vi "Write DAQ FIFO.vi"(6 "FIFO Timestamps":T2, 8 "error in (no error)":errorcluster, 9 "Timeout (ms)":i32, 10 "Data In":T1[](array[typedef]), 11 "CIFFIFO in":refnum<class "CIF_CIPC_Fifo_DAQ.lvclass">) -> (0 "error out":errorcluster, 1 "timed out?":bool, 2 "Data Out":T1[](array[typedef]), 3 "CIFFIFO out":refnum<class "CIF_CIPC_Fifo_DAQ.lvclass">)   [LabVIEW 2021, in "CIF_CIPC_Fifo_DAQ.lvclass"]
uses:
  CIF_CIPC_Fifo_DAQ.lvclass
  ChannelCommon/typedef/TimeStamps.ctl
  D:/dev/Packages/CIF_Channels_Core/src/CIPC_Channels/CIF_CIPC_Chan/CIF_CIPC_Chn.lvclass
  D:/dev/Packages/CIF_Channels_Core/src/CIFChannels/CIFChannels.lvclass
  ChannelCommon/typedef/Datatype Waveform.ctl
  CIFChannels/CIFChannels.lvclass/CIFChannels.ctl
  CIF_CIPC_Chan/CIF_CIPC_Chn.lvclass/CIF_CIPC_Chn.ctl
  <vilib>/CIF Foundation/CIF Utilities/Statistics/I64/Stats_I64_CIF_U.lvclass/Stats_I64_CIF_U.ctl
  CIF_CIPC_Chan/Accessors/Read Buffer Configuration.vi
  CIF_CIPC_Chan/SubVIs/Check Writer Backpressure.vi/7796537b-0e69-421b-96bb-30a861203fb6.vi
  CIFChannels/Accessors/Read FIFO Backpressure.vi
  CIFChannels/Utilities/Update Channel Benchmark.vi
  SubVIs/Core Write DAQ FIFO.vi/1bad10da-a98b-49ee-b03a-18b497e396df.vi
  SubVIs/Core Write DAQ FIFO.vi/70f860b1-5d4a-43dc-b0c2-c9446e8447f7.vi
  CIF_CIPC_Chan/Accessors/Read CIPC Channel.vi
  SubVIs/Write One DAQ Waveform.vi
  CIFChannels/Utilities/Create Flattened FIFO Header.vi
  CIF_CIPC_Chan/SubVIs/Write FIFO Header to CIPC.vi/2516c5c4-bcd6-4eab-a054-fa3d4f1376bc.vi
  CIF_CIPC_Chan/SubVIs/Check Writer Backpressure.vi/7796537b-0e69-421b-96bb-30a861203fb6.vi/3d5c1244-b460-4622-96d1-ee1e369932ac.vi
  <vilib>/CIF Foundation/CIF CIPC/Utilities/Get Size.vi
  CIF_CIPC_Chan/SubVIs/Check Writer Backpressure.vi/7796537b-0e69-421b-96bb-30a861203fb6.vi/b3361ac9-0b85-4d75-8feb-76d028d0c03f.vi
  <vilib>/CIF Foundation/CIF CIPC/SubVIs/Get Element Write Position.vi
  <vilib>/CIF Foundation/CIF Utilities/Statistics/I64/X1 minus X0.vi
  <vilib>/CIF Foundation/CIF Utilities/Time/System Time/Get System Time.vi
  SubVIs/Write One DAQ Waveform.vi/48238f55-1c09-49b5-9564-fcee243396a4.vi
  SubVIs/Write One DAQ Waveform.vi/652cb35b-0a2d-4ac6-8d88-471c3b57ed63.vi
  SubVIs/Write One DAQ Waveform.vi/5604da8b-43be-42ee-b0d1-5bd59e62de3d.vi
  SubVIs/Write One DAQ Waveform.vi/489ce88f-d13b-4e3d-8a44-beac6fbb575f.vi
  ChannelCommon/Utilities/Flatten Header.vi
  CIFChannels/Utilities/Update FIFO Header.vi
  ChannelCommon/Utilities/Add Header Bytes.vi
  <vilib>/CIF Foundation/CIF CIPC/SubVIs/Check Error.vi
  <vilib>/CIF Foundation/CIF CIPC/SubVIs/Notify Of New Write.vi
  <vilib>/CIF Foundation/CIF CIPC/SubVIs/Get dll Path.vi
  <vilib>/CIF Foundation/CIF CIPC/SubVIs/Wait For N Elements Available.vi
  <vilib>/CIF Foundation/CIF CIPC/SubVIs/Get Element Read Position.vi
  <vilib>/CIF Foundation/CIF CIPC/SubVIs/Set Element Read Position.vi
  <vilib>/CIF Foundation/CIF Utilities/Statistics/I64/X1 minus X0.vi/dfabcf33-0dbc-4041-80a5-3dc0c86d2989.vi
  <vilib>/CIF Foundation/CIF Utilities/Time/System Time/LabVIEW Time to TAI Time.vi
  <vilib>/CIF Foundation/CIF Utilities/DataTypes/Flatten Unflatten/Flatten U64.vi
  <vilib>/CIF Foundation/CIF Utilities/DataTypes/Flatten Unflatten/Flatten I64.vi
  <vilib>/CIF Foundation/CIF Utilities/Statistics/I64/X1 minus X0.vi/dfabcf33-0dbc-4041-80a5-3dc0c86d2989.vi/9eb60a9a-770f-4d2d-8b3f-8465c267ecc9.vi
  CIF_CIPC_Chan/CIF_CIPC_Chn.lvclass
  <vilib>/Utility/error.llb/Trim Whitespace.vi
  <vilib>/Utility/error.llb/Error Cluster From Error Code.vi
  <vilib>/CIF Foundation/CIF CIPC/SubVIs/Get Element Info Variant.vi
  ChannelCommon/ChannelCommon.lvlib
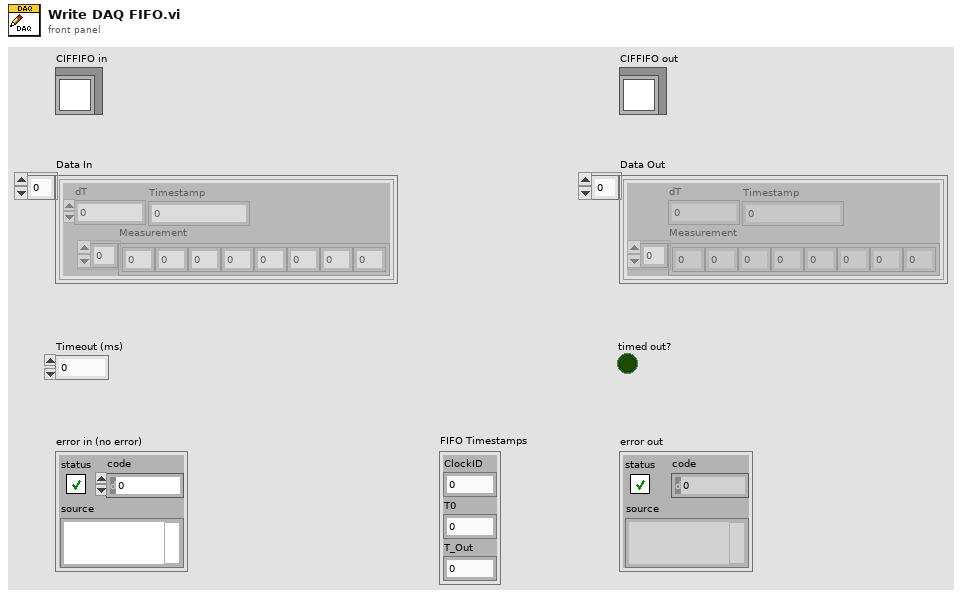
[diagram p1: front panel]
types:
  T1 = typedef "ChannelCommon.lvlib/Datatype Waveform.ctl" = cluster{"Measurement":dbl[], "dT":dbl, "Timestamp":i64}
  T2 = typedef "ChannelCommon.lvlib/TimeStamps.ctl" = cluster{"ClockID":u8, "T0":i64, "T_Out":i64}
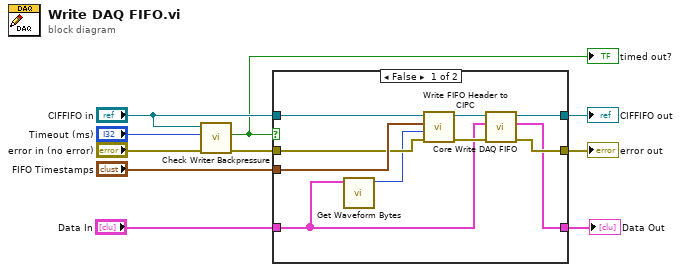
[diagram p0: block diagram]
diagram:
  n1 = call "Check Writer Backpressure.vi"("error in (no error)"="error in (no error)", "Timeout (ms)"="Timeout (ms)", "CIF_CIPC_Chn in"="CIFFIFO in") -> ("error out"=w10:errorcluster, "timed out?"=w5:bool)  [unwired: 7 in]
  "timed out?" <- w5
  n2 = case shown="False" w5 {
    tunnel: [w20 w23] -> w3
    tunnel: [w19 w22] -> w4
    tunnel: "FIFO Timestamps" -> [w18 _]
    tunnel: "Data In" -> [w11 w21]
    tunnel: "CIFFIFO in" -> [w15 w22]
    tunnel: w10 -> [w14 w23]
    tunnel: [w13 w21] -> w1
    frame False {
      n3 = call "Get Waveform Bytes.vi"("Waveforms"=w11) -> ("Bytes"=w12:i32)  [unwired: 10 in]
      n4 = call "Write FIFO Header to CIPC.vi"("error in (no error)"=w14, "Payload Length (bytes)"=w12, "FIFO Timestamps"=w18, "CIF_CIPC_Chn in"=w15) -> ("error out"=w16:errorcluster, "CIF_CIPC_Chn out"=w17:refnum<class "CIF_CIPC_Fifo_DAQ.lvclass">)  [unwired: 6 in]
      n5 = call "Core Write DAQ FIFO.vi"("error in (no error)"=w16, "Data In"=w11, "CIFFIFO in"=w17) -> ("error out"=w20:errorcluster, "Data Out"=w13:T1[], "CIFFIFO out"=w19:refnum<class "CIF_CIPC_Fifo_DAQ.lvclass">)  [unwired: 6 in]
    }
    frame True {
    }
  }
  "error out" <- w3
  "CIFFIFO out" <- w4
  "Data Out" <- w1
